vi "Do.vi"(8 "error in (no error)":errorcluster, 10 "Actor in":refnum<class "Actor.lvclass">, 11 "Addition Result Msg":refnum<class "Addition Result Msg.lvclass">) -> (0 "error out":errorcluster, 2 "Actor out":refnum<class "Actor.lvclass">)   [LabVIEW 2015, in "Addition Result Msg.lvclass"]
doc: "(<B>Filename</B>: Actor Framework.lvlib:Message.lvclass:Do.vi)\n\nDefines what a message does when it is received by an actor. Generally, a message instructs an actor to invoke one of its methods. By default, this method does nothing. A child class must override it to define behavior. Create a child class by using the Actor Framework Message Maker dialog box."
uses:
  Addition Result Msg.lvclass
  <vilib>/ActorFramework/Actor/Actor.lvclass
  Calculator Actor Class/Calculator Actor.lvclass
  Addition Result Msg.lvclass/Addition Result Msg.ctl
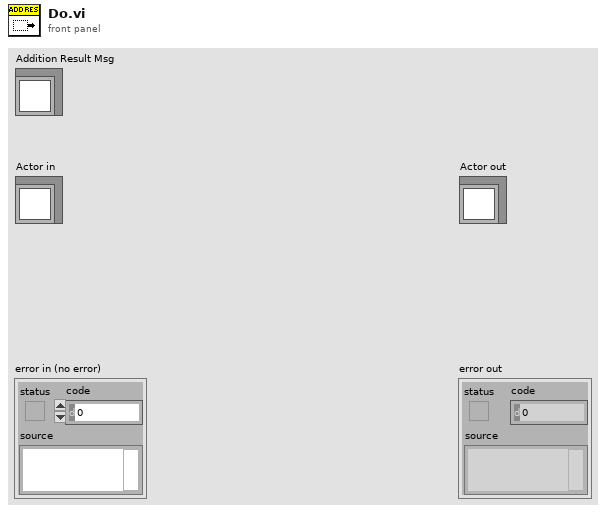
[diagram p1: front panel]
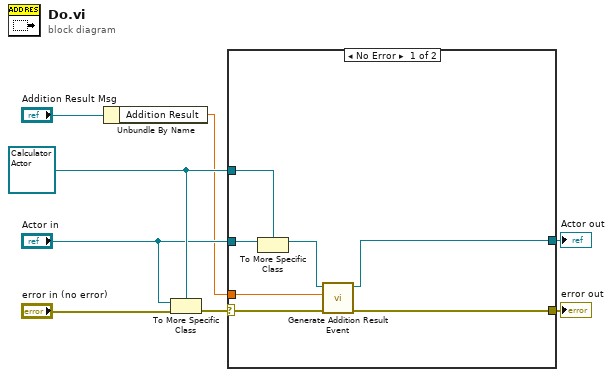
[diagram p0: block diagram]
diagram:
  w5 = refnum<class "Calculator Actor.lvclass"> refnum ("Calculator Actor in")
  n1 = Unbundle By Name("Addition Result Msg") -> ("Addition Result"=w3:dbl)
  n2 = To More Specific Class(target class=w5, reference="Actor in", error in="error in (no error)") -> (error out=w7:errorcluster)  [unwired: 1 out]
  n3 = case shown="No Error" w7 {
    selector: w7 -> [w13 w16]
    tunnel: w5 -> [w15 _]
    tunnel: "Actor in" -> [w14 w17]
    tunnel: w3 -> [w11 _]
    tunnel: [w10 w17] -> w2
    tunnel: [w9 w16] -> w1
    frame No Error {
      n4 = To More Specific Class(target class=w15, reference=w14) -> (specific class reference=w12:refnum<class "Calculator Actor.lvclass">)  [unwired: 1 in, 1 out]
      n5 = call "Generate Addition Result Event.vi"("error in (no error)"=w13, "Addition Result"=w11, "Calculator Actor in"=w12) -> ("error out"=w9:errorcluster, "Calculator Actor out"=w10:refnum<class "Calculator Actor.lvclass">)  [unwired: 7 in]
    }
    frame Error {
    }
  }
  "error out" <- w1
  "Actor out" <- w2
